vi "SMO_Demo.TestLauncher.vi"() -> ()   [LabVIEW 2016]
uses:
  <vilib>/JKI/JKI SMO/SMO/Typedefs/SMOState --Enum.ctl
  Typedefs/PublicEvents--SMO_Demo.PublicEvent.ctl
  SMO_Demo.lvclass
  C:/Program Files (x86)/National Instruments/LabVIEW 2016/vi.lib/JKI/JKI SMO/SMO/SMO.lvclass
  <vilib>/JKI/JKI SMO/SMO/SMO.lvclass
panel:
  in  "PublicMethod":string
  out "PublicEvent":T1
  out "SMO State":T2
  out "error out":errorcluster
  in  "Stop":bool
  # "Basic SMO Test Launcher"
  # "For instructions on how to use the JKI State Machine Objects, examples and video tutorials, visit:\nhttp://jki.net/state-machine-objects/\n\nJKI State Machine Objects™\nhttp://jki.net/state-machine-objects/\nCopyright (C) 2005-2015, JKI <info@jki.net>\nALL RIGHTS RESERVED"
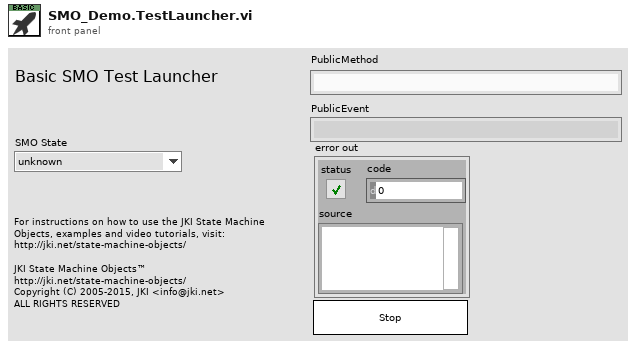
[diagram p1: front panel]
types:
  T1 = typedef "SMO_Demo.lvclass/PublicEvents--SMO_Demo.PublicEvent.ctl" = string
  T2 = typedef "SMO.lvclass/SMOState --Enum.ctl" = enum16{"unknown", "Created", "Started", "Stopped"}
  T3 = typedef "SMO.lvclass/Public Events.ctl" = cluster{"Error":refnum<user-event>, "State":refnum<user-event>, "Reserve State":refnum<user-event>}
  T4 = typedef "SMO_Demo.lvclass/PublicEvents--Cluster.ctl" = cluster{"PublicEvent":refnum<user-event>}
  T5 = cluster{"Event Registration Refnum":refnum<event-registration>}
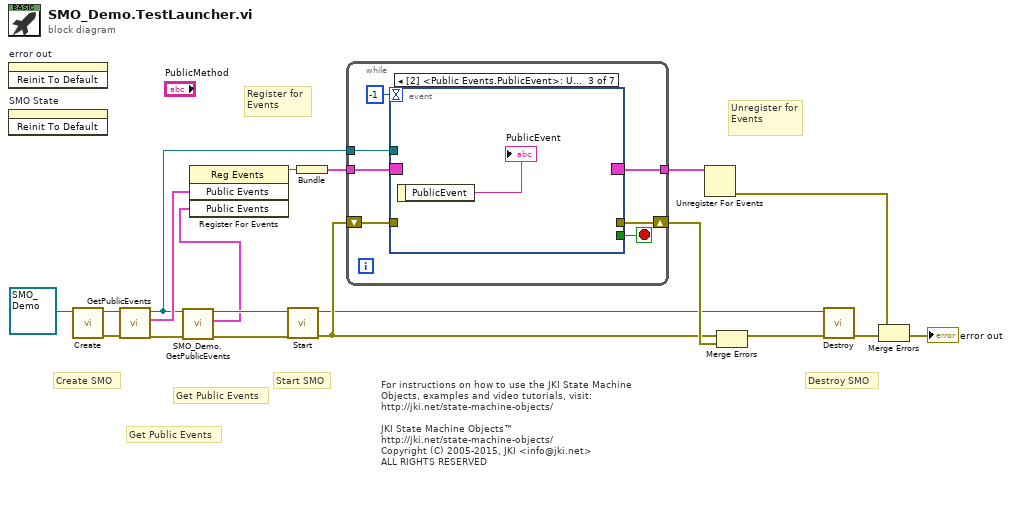
[diagram p0: block diagram]
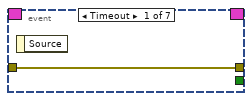
[diagram p2: hidden frame]
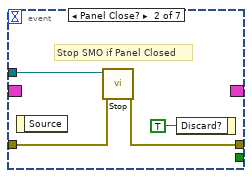
[diagram p3: hidden frame]
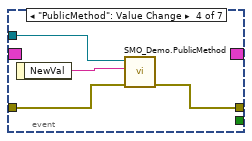
[diagram p4: hidden frame]
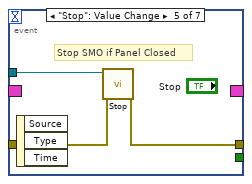
[diagram p5: hidden frame]
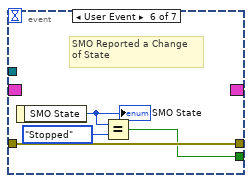
[diagram p6: hidden frame]
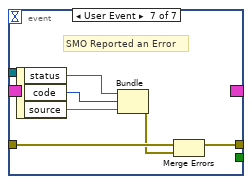
[diagram p7: hidden frame]
diagram:
  # "Get Public Events"
  # "For instructions on how to use the JKI State Machine Objects, examples and video tutorials, visit:\nhttp://jki.net/state-machine-objects/\n\nJKI State Machine Objects™\nhttp://jki.net/state-machine-objects/\nCopyright (C) 2005-2015, JKI <info@jki.net>\nALL RIGHTS RESERVED"
  # "Get Public Events"
  # "Start SMO"
  # "Destroy SMO"
  # "Create SMO"
  # "Unregister for Events"
  # "Register for Events"
  n1 = invoke on="error out" class="Clust (strict)" method="Reinit To Default"() -> ()  [unwired: 3 in, 3 out]
  n2 = invoke on="SMO State" class="Enum (strict)" method="Reinit To Default"() -> ()  [unwired: 3 in, 3 out]
  n3 = call <vilib>:"Create.vi"("SMO"=refnum<class "SMO_Demo.lvclass"> refnum ("SMO.Template.lvclass")) -> ("error out"=w8:errorcluster, "SMO out"=w9:refnum<class "SMO_Demo.lvclass">)  [unwired: 8 in, 1 out]
  n4 = call <vilib>:"GetPublicEvents.vi"("error in (no error)"=w8, "SMO"=w9) -> ("error out"=w4:errorcluster, "Public Events"=w7:T3, "SMO out"=w5:refnum<class "SMO_Demo.lvclass">)  [unwired: 7 in]
  n5 = call "SMO_Demo.GetPublicEvents.vi"("error in (no error)"=w4, "SMO_Demo"=w5) -> ("error out"=w3:errorcluster, "Public Events"=w1:T4, "SMO_Demo out"=w2:refnum<class "SMO_Demo.lvclass">)  [unwired: 7 in]
  n6 = register-events(w7, w1) -> (reference out=w6:refnum<event-registration>)  [unwired: 2 in, 1 out]
  n7 = call <vilib>:"Start.vi"("error in (no error)"=w3, "SMO"=w2) -> ("error out"=w12:errorcluster, "SMO out"=w10:refnum<class "SMO_Demo.lvclass">)  [unwired: 8 in]
  n8 = Bundle("Event Registration Refnum"=w6) -> (w18:T5)  [unwired: 1 in]
  n9 = while {
    shift-right: [w25] -> w17
    shift-left: w12 -> [w24]
    tunnel: w18 -> [w23]
    tunnel: [w22] -> w19
    tunnel: w5 -> [w21]
    stop <- w26 stop-if-true
    n10 = event shown="[2] <Public Events.PublicEvent>: User Event" {
      selector: w23 -> [_ _ _ _ _ _ _]
      dyn-events: [_ _ _ _ _ _ _] -> w22
      timeout: -1 -> [_ _ _ _ _ _ _]
      tunnel: [_ _ _ _ _ w40 _] -> w26
      tunnel: w21 -> [_ w31 _ w36 w39 _ _]
      tunnel: [w27 w30 _ w34 w38 w43 w47] -> w25
      tunnel: w24 -> [w27 w29 _ w35 w37 w43 w45]
      event Timeout {
        n11 = event-data() -> ()  [unwired: 1 in, 1 out]
      }
      event Panel Close? {
        # "Stop SMO if Panel Closed"
        n12 = event-data() -> ()  [unwired: 1 in, 1 out]
        n13 = call <vilib>:"Stop.vi"("error in (no error)"=w29, "SMO"=w31) -> ("error out"=w30:errorcluster)  [unwired: 8 in, 1 out]
        n14 = event-data("Discard?"=TRUE ("OK")) -> ()  [unwired: 1 in, 1 out]
      }
      event User Event {
        n15 = event-data() -> ("PublicEvent"=→"PublicEvent":T1)  [unwired: 1 in]
      }
      event "PublicMethod": Value Change {
        n16 = event-data() -> ("NewVal"=w33:string)  [unwired: 1 in]
        n17 = call "SMO_Demo.PublicMethod.vi"("error in (no error)"=w35, "PublicMethod"=w33, "SMO_Demo"=w36) -> ("error out"=w34:errorcluster)  [unwired: 7 in, 1 out]
      }
      event "Stop": Value Change {
        # "Stop SMO if Panel Closed"
        n18 = event-data() -> ()  [unwired: 1 in, 3 out]
        n19 = call <vilib>:"Stop.vi"("error in (no error)"=w37, "SMO"=w39) -> ("error out"=w38:errorcluster)  [unwired: 8 in, 1 out]
      }
      event User Event {
        # "SMO Reported a Change\nof State"
        n20 = event-data() -> ("SMO State"=w42:T2)  [unwired: 1 in]
        "SMO State" <- w42
        n21 = Equal?(x=w42, y=SMOState_--Enum."Stopped") -> (x = y?=w40:bool)
      }
      event User Event {
        # "SMO Reported an Error"
        n22 = event-data() -> ("status"=w46:bool, "code"=w49:i32, "source"=w48:string)  [unwired: 1 in]
        n23 = Bundle("status"=w46, "code"=w49, "source"=w48) -> (w44:errorcluster)  [unwired: 1 in]
        n24 = Merge Errors(w45, w44) -> (w47:errorcluster)
      }
    }
  }
  n25 = Unregister For Events(event registration refnum=w19) -> (error out=w16:errorcluster)  [unwired: 1 in]
  n26 = Merge Errors(w12, w17) -> (w11:errorcluster)
  n27 = call <vilib>:"Destroy.vi"("error in (no error)"=w11, "SMO"=w10) -> ("error out"=w14:errorcluster)  [unwired: 9 in]
  n28 = Merge Errors(w16, w14) -> (→"error out":errorcluster)
